vi "G#Object_GetClassType.vi"(1 "class path":path, 5 "error in (no error)":errorcluster) -> (14 "reference out":refnum<class "G#Object.lvclass">, 19 "error out":errorcluster)   [LabVIEW 2020, in "G#Object.lvclass"]
doc: "Returns an invalid G#Object of the type specified by the class path. Use this VI to dynamically select class type and load it into memory."
uses:
  <vilib>/addons/_AddQ/G#Object/G#Object.lvclass
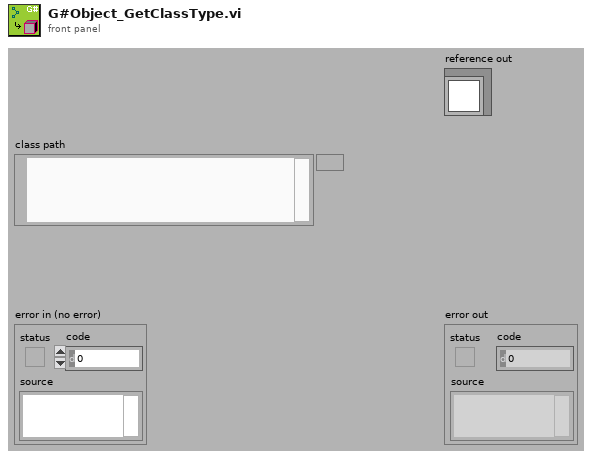
[diagram p1: front panel]
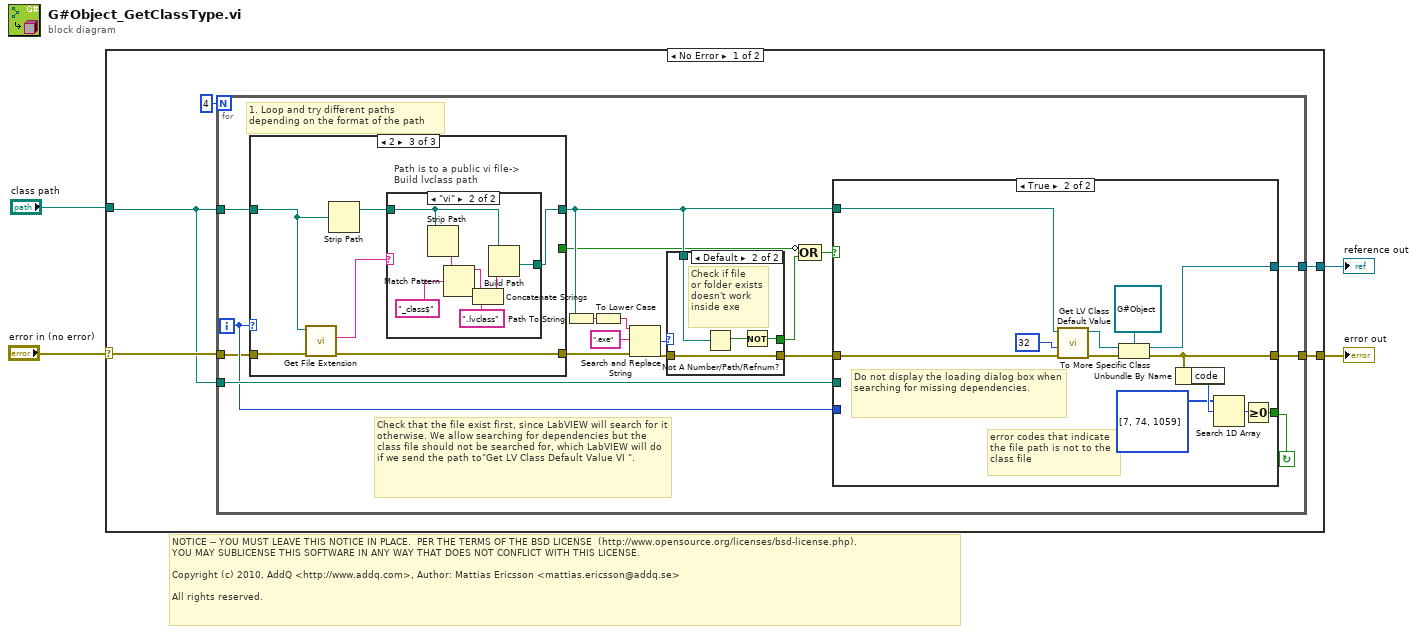
[diagram p0: block diagram]
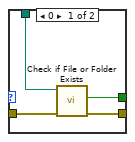
[diagram p2: hidden frame]
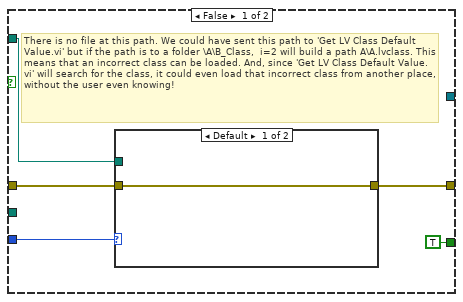
[diagram p3: hidden frame]
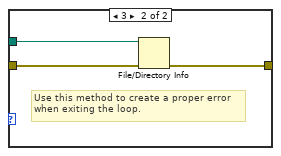
[diagram p4: hidden frame]
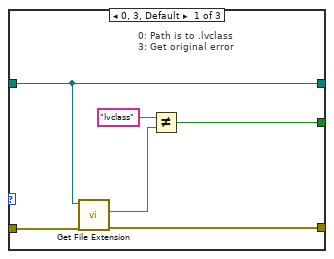
[diagram p5: hidden frame]
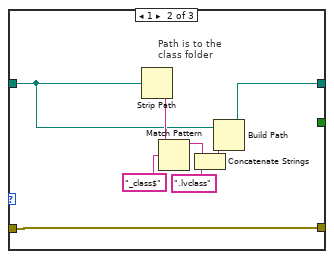
[diagram p6: hidden frame]
diagram:
  # "NOTICE -- YOU MUST LEAVE THIS NOTICE IN PLACE.  PER THE TERMS OF THE BSD LICENSE  (http://www.opensource.org/licenses/bsd-license.php).\nYOU MAY SUBLICENSE THIS SOFTWARE IN ANY WAY THAT DOES NOT CONFLICT WITH THIS LICENSE.\n\nCopyright (c) 2010, AddQ <http://www.addq.com>, Author: Mattias Ericsson <mattias.ericsson@addq.se>\n\nAll rights reserved."
  n1 = case shown="No Error" "error in (no error)" {
    selector: "error in (no error)" -> [w9 w84]
    tunnel: [w6 w84] -> w3
    tunnel: [w8 _] -> w2
    tunnel: "class path" -> [w5 _]
    frame No Error {
      n2 = for {
        N: 4 -> [_]
        tunnel: w5 -> [w27]
        tunnel: [w26] -> w8
        tunnel: w9 -> [w14]
        tunnel: [w24] -> w6
        tunnel: w5 -> [w22]
        i -> [w21]
        stop <- w25 continue-if-true
        # "Check that the file exist first, since LabVIEW will search for it otherwise. We allow searching for dependencies but the class file should not be searched for, which LabVIEW will do if we send the path to\"Get LV Class Default Value VI \"."
        # "1. Loop and try different paths\ndepending on the format of the path"
        n3 = case shown="2" w21 {
          tunnel: w27 -> [w60 w64 w71]
          tunnel: [w60 w65 w76] -> w20
          tunnel: w14 -> [w62 w63 w74]
          tunnel: [w61 w63 w75] -> w13
          tunnel: [w57 _ _] -> w12
          frame 0, 3, Default {
            # "0: Path is to .lvclass\n3: Get original error"
            n4 = call <vilib>:"Get File Extension.vi"("error in (no error)"=w62, "file"=w60) -> ("error out"=w61:errorcluster, "lowercase file extension"=w59:string)  [unwired: 5 in, 3 out]
            n5 = Not Equal?(x="lvclass", y=w59) -> (x != y?=w57:bool)
          }
          frame 1 {
            # "Path is to the \nclass folder"
            n6 = Strip Path(path=w64) -> (name=w70:string)  [unwired: 1 out]
            n7 = Match Pattern(string=w70, regular expression="_class$") -> (before substring=w68:string)  [unwired: 1 in, 3 out]
            n8 = Concatenate Strings(w68, ".lvclass" ("string")) -> (w66:string)
            n9 = Build Path(base path=w64, name or relative path=w66) -> (appended path=w65:path)
          }
          frame 2 {
            # "Path is to a public vi file->\nBuild lvclass path"
            n10 = call <vilib>:"Get File Extension.vi"("error in (no error)"=w74, "file"=w71) -> ("error out"=w75:errorcluster, "lowercase file extension"=w73:string)  [unwired: 5 in, 3 out]
            n11 = Strip Path(path=w71) -> (stripped path=w72:path)  [unwired: 1 out]
            n12 = case shown="\"vi\"" w73 {
              tunnel: [_ w78] -> w76
              tunnel: w72 -> [_ w77]
              frame Default {
                # "not a vi file path"
              }
              frame "vi" {
                n13 = Strip Path(path=w77) -> (name=w83:string)  [unwired: 1 out]
                n14 = Match Pattern(string=w83, regular expression="_class$") -> (before substring=w81:string)  [unwired: 1 in, 3 out]
                n15 = Concatenate Strings(w81, ".lvclass" ("string")) -> (w79:string)
                n16 = Build Path(base path=w77, name or relative path=w79) -> (appended path=w78:path)
              }
            }
          }
        }
        n17 = Path To String(path=w20) -> (string=w19:string)
        n18 = To Lower Case(string=w19) -> (all lower case string=w16:string)
        n19 = Search and Replace String(input string=w16, search string=".exe", error in=w13) -> (number of replacements=w15:i32, error out=w17:errorcluster)  [unwired: 5 in, 2 out]
        n20 = case shown="Default" w15 {
          tunnel: [w31 w35] -> w23
          tunnel: w20 -> [w30 w34]
          tunnel: [w29 w33] -> w11
          tunnel: w17 -> [w28 w35]
          frame 0 {
            n21 = call <vilib>:"Check if File or Folder Exists.vi"("error in (no error)"=w28, "path"=w30) -> ("error out"=w31:errorcluster, "file or folder exists?"=w29:bool)  [unwired: 7 in, 1 out]
          }
          frame Default {
            # "Check if file\nor folder exists\ndoesn't work\ninside exe"
            n22 = Not A Number/Path/Refnum?(number/path/refnum=w34) -> (NaN/Path/Refnum?=w32:bool)
            n23 = Not(x=w32) -> (.not. x?=w33:bool)
          }
        }
        n24 = Compound Arithmetic op=OR(invert w12, w11) -> (w10:bool)
        n25 = case shown="True" w10 {
          tunnel: [_ w52] -> w26
          tunnel: [TRUE w48] -> w25
          tunnel: [w38 w47] -> w24
          tunnel: w20 -> [w36 w46]
          tunnel: w23 -> [w39 w45]
          tunnel: w22 -> [_ _]
          tunnel: w21 -> [w37 _]
          frame False {
            # "There is no file at this path. We could have sent this path to 'Get LV Class Default Value.vi' but if the path is to a folder \\A\\B_Class,  i=2 will build a path A\\A.lvclass. This means that an incorrect class can be loaded. And, since 'Get LV Class Default Value.vi' will search for the class, it could even load that incorrect class from another place, without the user even knowing!"
            n26 = case shown="Default" w37 {
              tunnel: w39 -> [w41 w44]
              tunnel: [w41 w43] -> w38
              tunnel: w36 -> [_ w42]
              frame Default {
              }
              frame 3 {
                # "Use this method to create a proper error\nwhen exiting the loop."
                n27 = File/Directory Info(path=w42, error in=w44) -> (error out=w43:errorcluster)  [unwired: 6 out]
              }
            }
          }
          frame True {
            # "Do not display the loading dialog box when searching for missing dependencies."
            # "error codes that indicate\nthe file path is not to the\nclass file"
            n28 = call <vilib>:"Get LV Class Default Value.vi"("error in (no error)"=w45, "options"=u32 32, "class path"=w46) -> ("error out"=w53:errorcluster, "object"=w54:refnum<class>)  [unwired: 7 in]
            n29 = To More Specific Class(target class=refnum<class "G#Object.lvclass"> refnum ("reference out"), reference=w54, error in=w53) -> (specific class reference=w52:refnum<class "G#Object.lvclass">, error out=w47:errorcluster)
            n30 = Unbundle By Name(w47) -> ("code"=w51:i32)
            n31 = Search 1D Array(1D array=i32[] [7, 74, 1059], element=w51) -> (index of element=w49:i32)  [unwired: 1 in]
            n32 = Greater Or Equal To 0?(x=w49) -> (x >= 0?=w48:bool)
          }
        }
      }
    }
    frame Error {
    }
  }
  "error out" <- w3
  "reference out" <- w2
